vi "RES_V_T.vi"(10 "Channel":T1(ring), 11 "VISA Refnum in":refnum<visa-resource-name>) -> (2 "Numeric 2":dbl, 3 "Numeric":dbl)   [LabVIEW 2020]
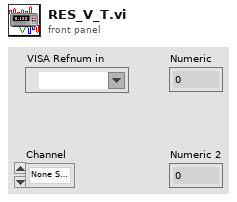
[diagram p1: front panel]
types:
  T1 = enum16{"None Selected", "1", "2", "3", "4", "5", "6", "7", "8", "9", "10", "11", "12", "13", "14", "15", "16"}
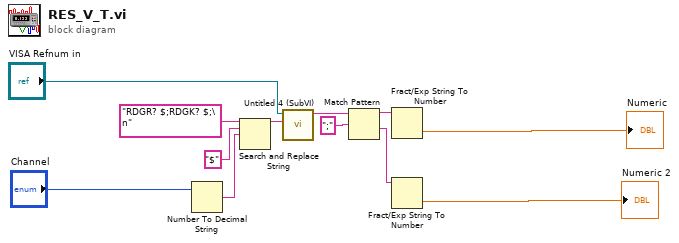
[diagram p0: block diagram]
diagram:
  n1 = Number To Decimal String(number="Channel") -> (decimal integer string=w4:string)  [unwired: 1 in]
  n2 = Search and Replace String(input string="RDGR? $;RDGK? $;\n" ("Command"), search string="$", replace string=w4) -> (result string=w6:string)  [unwired: 5 in, 3 out]
  n3 = call "Untitled 4 (SubVI).vi"("ID Query"=w6, "VISA Refnum in"="VISA Refnum in") -> ("read buffer"=w7:string)  [unwired: 9 in]
  n4 = Match Pattern(string=w7, regular expression=";") -> (before substring=w9:string, after substring=w10:string)  [unwired: 1 in, 2 out]
  n5 = Fract/Exp String To Number(string=w9) -> (number=→"Numeric":dbl)  [unwired: 3 in, 1 out]
  n6 = Fract/Exp String To Number(string=w10) -> (number=→"Numeric 2":dbl)  [unwired: 3 in, 1 out]
